vi "update nested DVR on caller.vi"(11 "Template in":refnum<class "Template.lvclass">) -> (0 "error out":errorcluster)   [LabVIEW 2020, in "Template.lvlib" / "Template.lvclass"]
uses:
  Template.lvclass
  C:/Program Files/National Instruments/LabVIEW 2020/vi.lib/ActorFramework/Actor/Actor.lvclass
  Template.lvclass/Template.ctl
  <vilib>/ActorFramework/Actor/Actor.lvclass/Actor.ctl
  Template Messages/update DVR pool from nested actors Msg/update DVR pool from nested actors Msg.lvclass/update DVR pool from nested actors Msg.ctl
  <vilib>/ActorFramework/Message Enqueuer/Message Enqueuer.lvclass/Message Enqueuer.ctl
  accessors/Read This Actor Number.vi
  <vilib>/ActorFramework/Message Enqueuer/Enqueue.vi
  Template Messages/update DVR pool from nested actors Msg/update DVR pool from nested actors Msg.lvclass
  C:/Program Files/National Instruments/LabVIEW 2020/vi.lib/ActorFramework/Message/Message.lvclass
  <vilib>/ActorFramework/Message Priority Queue/Priority Enqueue.vi
  <vilib>/ActorFramework/Actor/Actor.lvclass
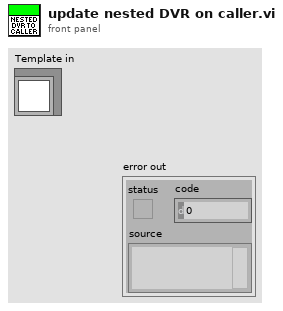
[diagram p1: front panel]
types:
  T1 = typedef "Template.lvlib/Template.lvclass/base actor queues.ctl" = cluster{"DVR Pool":refnum<queue>, "Actor's Data":refnum<queue>}
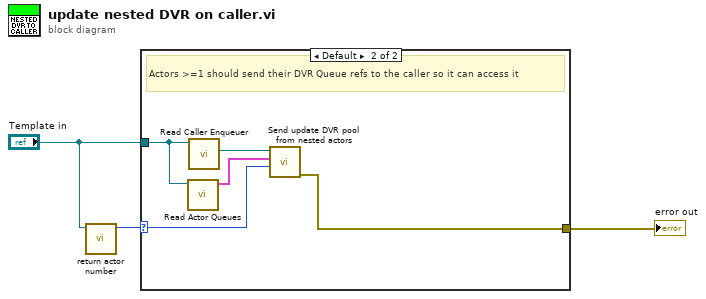
[diagram p0: block diagram]
diagram:
  n1 = call "return actor number.vi"("Template in"="Template in") -> ("Actor number"=w2:u32)  [unwired: 10 in]
  n2 = case shown="Default" w2 {
    selector: w2 -> [_ w5]
    tunnel: "Template in" -> [_ w7]
    tunnel: [_ w4] -> w1
    frame 0 {
      # "Actor 0 produces no data, so no need to send its DVR Queue ref"
    }
    frame Default {
      # "Actors >=1 should send their DVR Queue refs to the caller so it can access it"
      n3 = call "Read Actor Queues.vi"("Template in"=w7) -> ("Base Actor Queues"=w6:T1)  [unwired: 10 in]
      n4 = call <vilib>:"Read Caller Enqueuer.vi"("Actor"=w7) -> ("Caller Enqueuer"=w8:refnum<class "Message Enqueuer.lvclass">)  [unwired: 10 in]
      n5 = call "Send update DVR pool from nested actors.vi"("Actor number"=w5, "Base Actor Queues"=w6, "Message Enqueuer"=w8) -> ("error out"=w4:errorcluster)  [unwired: 7 in, 1 out]
    }
  }
  "error out" <- w1
